vi "NearestCentroid.vi"(8 "error in":errorcluster) -> (0 "error out":errorcluster, 3 "out":refnum<class "NearestCentroid.lvclass">)   [LabVIEW 2020]
doc: "Nearest centroid classifier.\n\n Each class is represented by its centroid, with test samples classified to\n the class with the nearest centroid.\n\n Read more in the :ref:`User Guide <nearest_centroid_classifier>`.\n\n Parameters\n ----------\n metric : str or callable\n The metric to use when calculating distance between instances in a\n feature array. If metric is a string or callable, it must be one of\n the options allowed by metrics.pairwise.pairwise_distances for its\n metric parameter.\n The centroids for the samples corresponding to each class is the point\n from which the sum of the distances (according to the metric) of all\n samples that belong to that particular class are minimized.\n If the \"manhattan\" metric is provided, this centroid is the median and\n for all other metrics, the centroid is now set to be the mean.\n\n .. versionchanged:: 0.19\n ``metric='precomputed'`` was deprecated and now raises an error\n\n shrink_threshold : float, default=None\n Threshold for shrinking centroids to remove features.\n\n Attributes\n ----------\n centroids_ : array-like of shape (n_classes, n_features)\n Centroid of each class.\n\n classes_ : array of shape (n_classes,)\n The unique classes labels.\n\n \nAvailable methods:\nFit\nPredict\nScore\nGet Attributes\nGet Params\nSet Params"
uses:
  NearestCentroid.lvclass
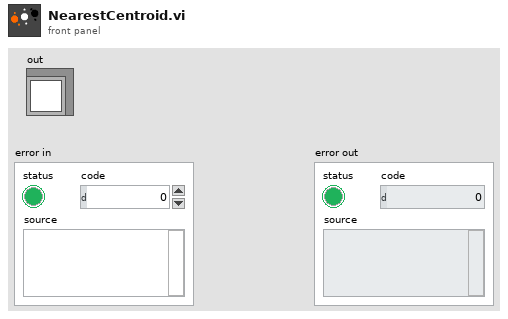
[diagram p1: front panel]
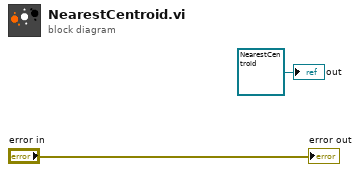
[diagram p0: block diagram]
diagram:
  "out" <- refnum<class "NearestCentroid.lvclass"> refnum ("model")
  "error out" <- "error in"
